vi "gen_text_data.vi"() -> ()   [LabVIEW 2019]
uses:
  results_data.ctl
  MainFGV/Settings/Advanced/AdvancedConfig.ctl
  <vilib>/Analysis/NI_AALPro.lvlib
panel:
  out "files_dir 2":path
  in  "min_band_width":dbl=400.0
  in  "files_dir":path
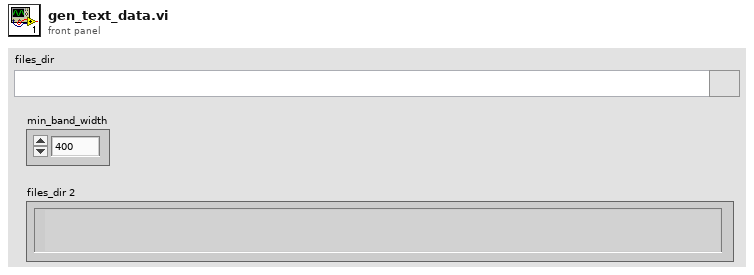
[diagram p1: front panel]
types:
  T1 = typedef "results_data.ctl" = cluster{"config":T2, "hammer":waveform(dbl), "acelerometers":waveform(dbl)[], "hammerIndex":i32}
  T2 = typedef "AdvancedConfig.ctl" = cluster{"rate":dbl, "duration":dbl, "thr":dbl, "preTrigger":dbl, "cutoff":dbl, "Filtro":enum16{"Desativado", "Passa banda", "Passa alta", "Passa baixa"}, "highPass":dbl, "lowPass":dbl, "updateTime":dbl}
  T3 = cluster{"seconds since 1Jan1904":timestamp, "data_out":T1}
  T4 = enum16{"open", "replace", "create", "open or create", "replace or create", "replace or create with confirmation"}
  T5 = cluster{"seconds since 1Jan1904":timestamp, "data_out":T1}[]
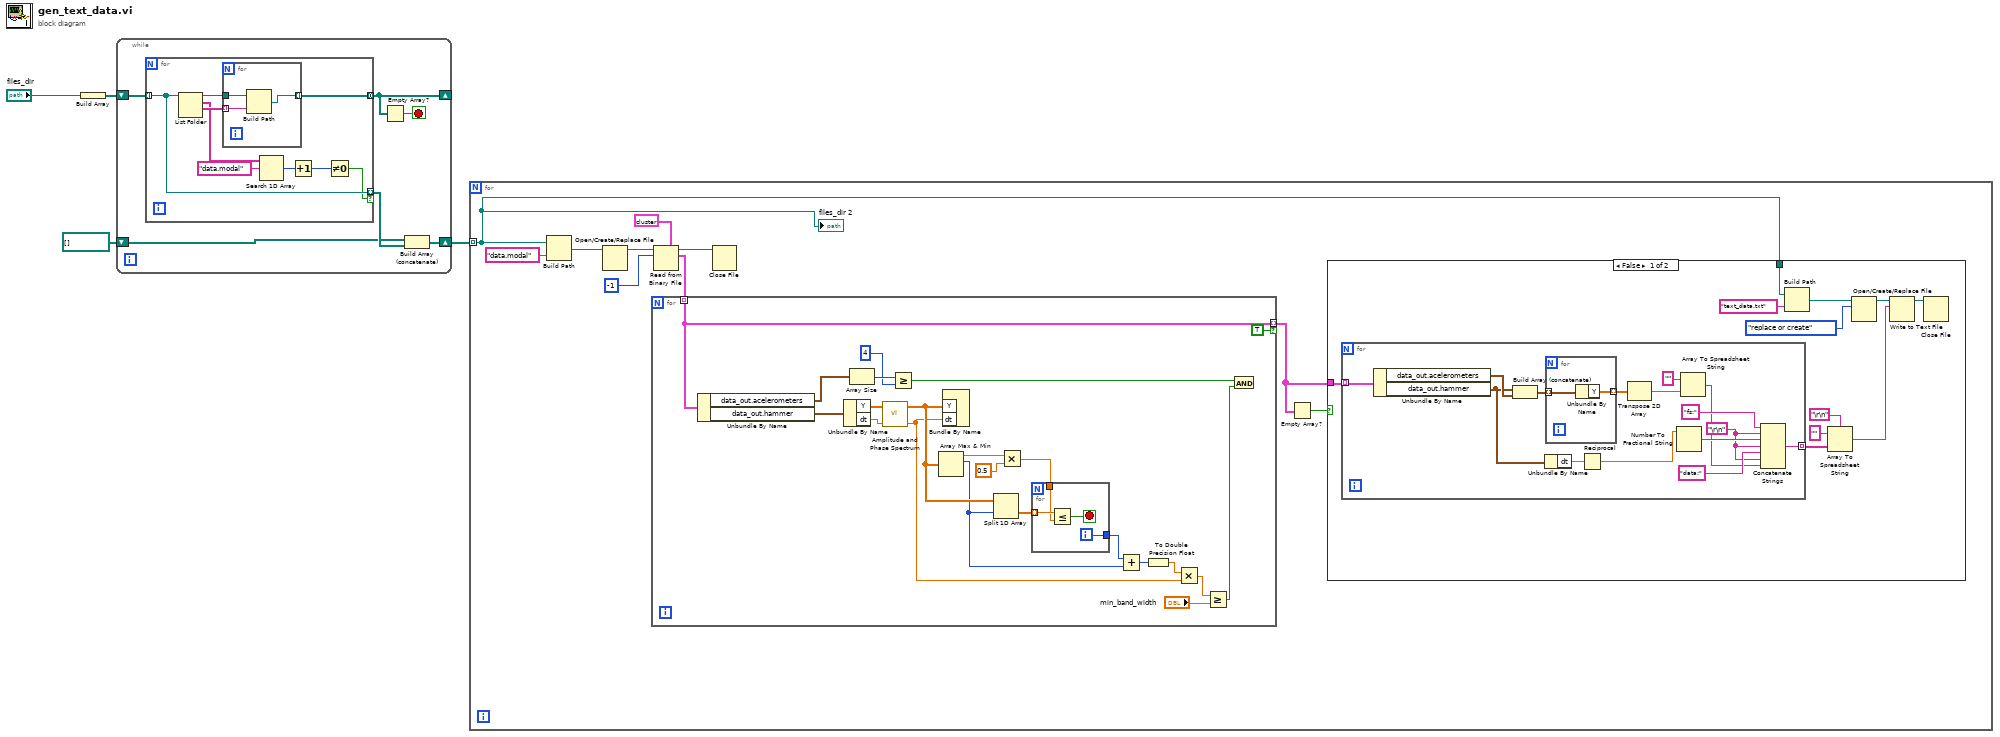
[diagram p0: block diagram]
diagram:
  n1 = Build Array("files_dir") -> (w3:path[])
  n2 = while {
    shift-right: [w7] -> _
    shift-left: w3 -> [w10]
    shift-right: [w8] -> w1
    shift-left: path[] [] -> [w5]
    stop <- w6 stop-if-true
    n3 = for {
      tunnel: w10 -> [w12] mode=indexing
      tunnel: [w17] -> w7 mode=concatenating
      tunnel: [w12] -> w9 mode=indexing if=w11
      n4 = List Folder(path=w12) -> (path out=w18:path, filenames=w16:string[], folder names=w19:string[])  [unwired: 3 in, 1 out]
      n5 = for {
        tunnel: w19 -> [w22] mode=indexing
        tunnel: w18 -> [w21]
        tunnel: [w20] -> w17 mode=indexing
        n6 = Build Path(base path=w21, name or relative path=w22) -> (appended path=w20:path)
      }
      n7 = Search 1D Array(1D array=w16, element="data.modal") -> (index of element=w14:i32)  [unwired: 1 in]
      n8 = Increment(x=w14) -> (x+1=w13:i32)
      n9 = Not Equal To 0?(x=w13) -> (x != 0?=w11:bool)
    }
    n10 = Empty Array?(array=w7) -> (empty?=w6:bool)
    n11 = Build Array (concatenate)(w5, w9) -> (w8:path[])
  }
  n12 = for {
    tunnel: w1 -> [w23] mode=indexing
    n13 = Build Path(base path=w23, name or relative path="data.modal") -> (appended path=w31:path)
    n14 = Open/Create/Replace File(file path (use dialog)=w31) -> (refnum out=w30:refnum<file>)  [unwired: 5 in, 2 out]
    n15 = Read from Binary File(5:T3 {"seconds since 1Jan1904"=timestamp(0 s since 1904-01-01), "data_out"={"config"={"rate"=0.0, "duration"=0.0, "thr"=0.0, "preTrigger"=0.0, "cutoff"=0.0, "Filtro"=enum."Desativado", "highPass"=0.0, "lowPass"=0.0, "updateTime"=0.0}, "hammer"={"t0"=timestamp(0 s since 1904-01-01), "dt"=1.0, "Y"=[]}, "acelerometers"=[], "hammerIndex"=0}} ("output cluster"), 10:-1 ("count (1)"), 11:w30) -> (2:w27:T5, 3:w28:refnum<file>)  [unwired: 3 in, 2 out]
    n16 = for {
      tunnel: w27 -> [w67] mode=indexing
      tunnel: [w67] -> w24 mode=indexing if=TRUE
      n17 = Unbundle By Name(w67) -> ("data_out.acelerometers"=w66:waveform(dbl)[], "data_out.hammer"=w82:waveform(dbl))
      n18 = Unbundle By Name(w82) -> ("Y"=w81:dbl[], "dt"=w80:dbl)
      n19 = Array Size(array=w66) -> (size(s)=w65:i32)
      n20 = call <vilib>:"Amplitude and Phase Spectrum.vi"("dt"=w80, "Signal (V)"=w81) -> ("df"=w70:dbl, "Amp Spectrum Mag (Vrms)"=w79:dbl[])  [unwired: 1 in, 1 out]
      n21 = Greater Or Equal?(x=w65, y=4) -> (x >= y?=w62:bool)
      n22 = Array Max & Min(array=w79) -> (max value=w78:dbl, max index (indices)=w73:i32)  [unwired: 2 out]
      n23 = Bundle By Name("Y"=w79, "dt"=w70) -> ()  [unwired: 1 in, 1 out]
      n24 = Split 1D Array(array=w79, index=w73) -> (second subarray=w76:dbl[])  [unwired: 1 out]
      n25 = Multiply(x=w78, y=0.5) -> (x*y=w75:dbl)
      n26 = for {
        tunnel: w76 -> [w86] mode=indexing
        tunnel: w75 -> [w85]
        tunnel: [w83] -> w74
        i -> [w83]
        stop <- w84 stop-if-true
        n27 = Less Or Equal?(x=w86, y=w85) -> (x <= y?=w84:bool)
      }
      n28 = Add(x=w74, y=w73) -> (x+y=w72:i32)
      n29 = To Double Precision Float(number=w72) -> (double precision float=w71:dbl)
      n30 = Multiply(x=w71, y=w70) -> (x*y=w69:dbl)
      n31 = Greater Or Equal?(x=w69, y="min_band_width") -> (x >= y?=w63:bool)
      n32 = And(x=w62, y=w63) -> ()  [unwired: 1 out]
    }
    n33 = Close File(refnum=w28) -> ()  [unwired: 1 in, 2 out]
    n34 = Empty Array?(array=w24) -> (empty?=w25:bool)
    n35 = case shown="False" w25 {
      tunnel: w24 -> [w43 _]
      tunnel: w23 -> [w40 _]
      frame False {
        n36 = for {
          tunnel: w43 -> [w58] mode=indexing
          tunnel: [w48] -> w42 mode=indexing
          w47 = "\r\n"
          n37 = Unbundle By Name(w58) -> ("data_out.acelerometers"=w57:waveform(dbl)[], "data_out.hammer"=w46:waveform(dbl))
          n38 = Build Array (concatenate)(w46, w57) -> (w56:waveform(dbl)[])
          n39 = Unbundle By Name(w46) -> ("dt"=w45:dbl)
          n40 = for {
            tunnel: w56 -> [w60] mode=indexing
            tunnel: [w59] -> w55 mode=indexing
            n41 = Unbundle By Name(w60) -> ("Y"=w59:dbl[])
          }
          n42 = Reciprocal(x=w45) -> (1/x=w44:dbl)
          n43 = Transpose 2D Array(2D array=w55) -> (transposed array=w53:dbl[][])
          n44 = Number To Fractional String(number=w44) -> (F-format string=w52:string)  [unwired: 3 in]
          n45 = Array To Spreadsheet String(array=w53, 3:"" ("format string")) -> (spreadsheet string=w49:string)  [unwired: 1 in]
          n46 = Concatenate Strings("fs:" ("string"), w47, w52, w47, "data:" ("string"), w47, w49) -> (w48:string)
        }
        n47 = Build Path(base path=w40, name or relative path="text_data.txt") -> (appended path=w38:path)
        n48 = Array To Spreadsheet String(delimiter (Tab)="\r\n", array=w42, 3:"" ("format string")) -> (spreadsheet string=w34:string)
        n49 = Open/Create/Replace File(file path (use dialog)=w38, operation (0:open)=T4."replace or create") -> (refnum out=w36:refnum<file>)  [unwired: 4 in, 2 out]
        n50 = Write to Text File(file (use dialog)=w36, text=w34) -> (refnum out=w35:refnum<file>)  [unwired: 2 in, 2 out]
        n51 = Close File(refnum=w35) -> ()  [unwired: 1 in, 2 out]
      }
      frame True {
      }
    }
    "files_dir 2" <- w23
  }
